vi "Error Converter (ErrCode or Status).vi"(8 "error in (no error)":errorcluster, 11 "error code":i32) -> (0 "error out":errorcluster)   [LabVIEW 2015, in "TPVG_DLL.lvlib"]
uses:
  TPVG_DLL.lvlib
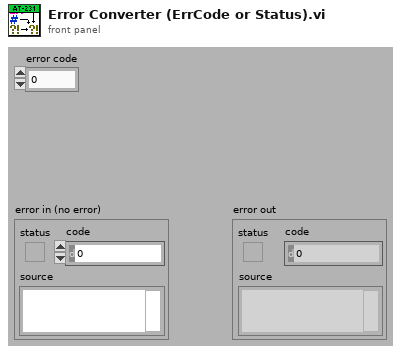
[diagram p1: front panel]
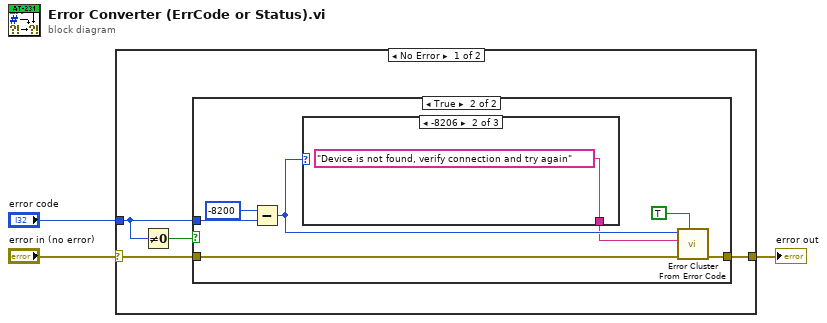
[diagram p0: block diagram]
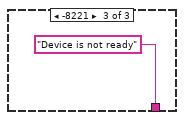
[diagram p4: hidden frame]
diagram:
  n1 = case shown="No Error" "error in (no error)" {
    selector: "error in (no error)" -> [w7 w18]
    tunnel: [w6 w18] -> w2
    tunnel: "error code" -> [w5 _]
    frame No Error {
      n2 = Not Equal To 0?(x=w5) -> (x != 0?=w4:bool)
      n3 = case shown="True" w4 {
        tunnel: w7 -> [w8 w15]
        tunnel: w5 -> [_ w12]
        tunnel: [w8 w14] -> w6
        frame False {
        }
        frame True {
          n4 = Subtract(x=-8200, y=w12) -> (x-y=w10:i32)
          n5 = case shown="-8206" w10 {
            tunnel: [_ "Device is not found, verify connection and try again" ("error message (\"\")") "Device is not ready" ("error message (\"\")")] -> w9
            frame 0, Default {
            }
            frame -8206 {
            }
            frame -8221 {
            }
          }
          n6 = call <vilib>:"Error Cluster From Error Code.vi"("show call chain? (False)"=TRUE, "error in (no error)"=w15, "error message (\"\")"=w9, "error code (0)"=w10) -> ("error out"=w14:errorcluster)  [unwired: 5 in]
        }
      }
    }
    frame Error {
    }
  }
  "error out" <- w2
